vi "Check if Reference.vi"(8 "error in (no error)":errorcluster, 11 "motor communication in":refnum<class "NI_Robotics_Motor Communication.lvclass">) -> (0 "error out":errorcluster, 1 "initialized?":bool, 2 "invalid refs?":bool, 3 "motor communication out":refnum<class "NI_Robotics_Motor Communication.lvclass">)   [LabVIEW 2017, in "NI_Robotics_Motor Communication.lvclass"]
uses:
  <vilib>/robotics/Actuation/Motor Communication/NI_Robotics_Motor Communication.lvclass
  <vilib>/robotics/Actuation/Motor Communication/NI_Robotics_Motor Communication.lvclass/NI_Robotics_Motor Communication.ctl
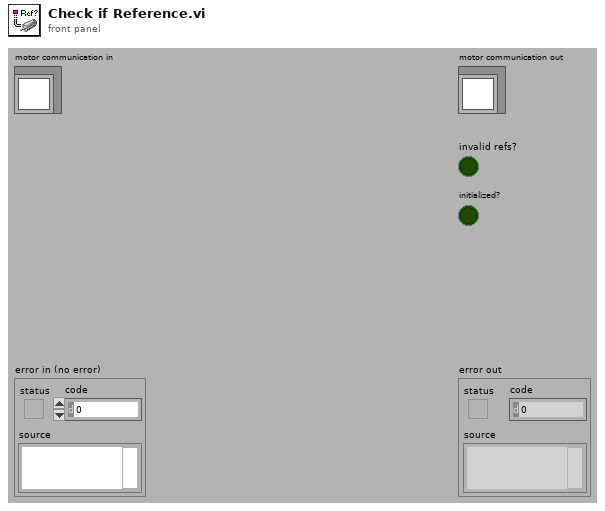
[diagram p1: front panel]
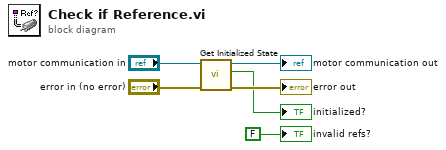
[diagram p0: block diagram]
diagram:
  n1 = call <vilib>:"Get Initialized State.vi"("error in (no error)"="error in (no error)", "motor communication in"="motor communication in") -> ("error out"=→"error out":errorcluster, "initialized"=→"initialized?":bool, "motor communication out"=→"motor communication out":refnum<class "NI_Robotics_Motor Communication.lvclass">)  [unwired: 7 in]
  "invalid refs?" <- FALSE ("reference?")
